vi "TSM SSC DAQmx Configure Sync Pulse Source PXI Trig.vi"(0 "DAQ TSM in":T1, 5 "source(PXI_Trig0)":string(combo)="PXI_Trig0", 11 "error in (no error)":errorcluster) -> (4 "DAQ TSM Out":T1, 15 "error out":errorcluster)   [LabVIEW 2020]
doc: "Specifies the terminal of the signal to use as the synchronization pulse. The synchronization pulse resets the clock dividers and the ADCs/DACs on the device."
uses:
  Pin Map/TSM DAQmx Multi-Task.ctl
  <vilib>/NI_TestStand_SemiconductorModule/NI_TestStand_Semiconductor_Module.lvlibp/PinMap/PinQueryContext/MultiplePinMultipleSessionQueryContext/MultiplePinMultipleSessionQueryContext.lvclass
  Pin Map/SSC DAQmx.ctl
  <resource>/objmgr/daqmx.rc
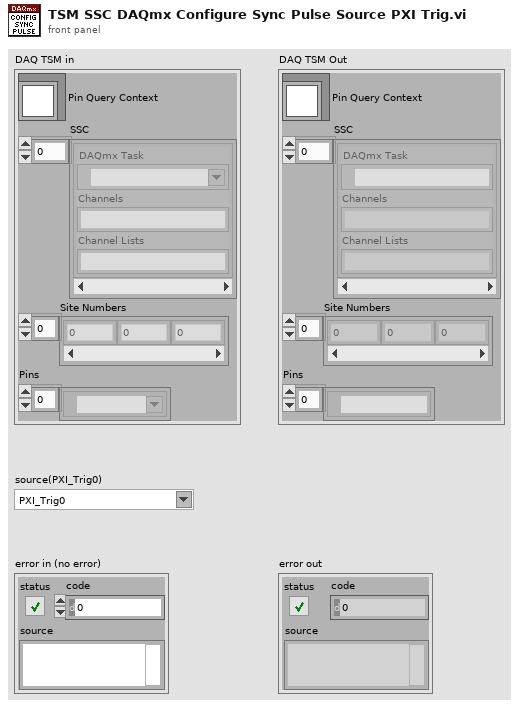
[diagram p1: front panel]
types:
  T1 = typedef "TSM DAQmx Multi-Task.ctl" = cluster{"Pin Query Context":refnum<class "MultiplePinMultipleSessionQueryContext.lvclass">, "SSC":T2[], "Site Numbers":i32[], "Pins":tag[]}
  T2 = typedef "SSC DAQmx.ctl" = cluster{"DAQmx Task ":refnum<k21>, "Channels":string, "Channel Lists":string}
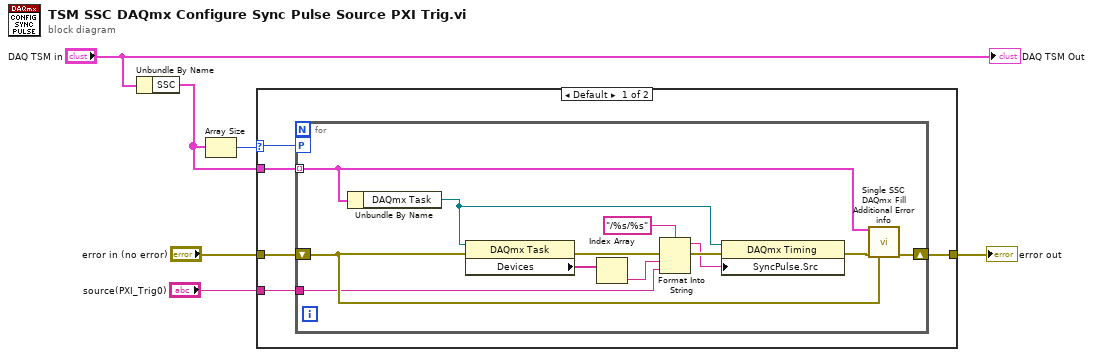
[diagram p0: block diagram]
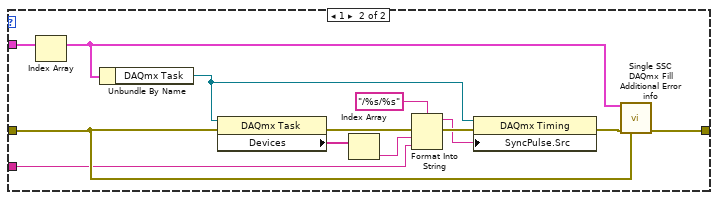
[diagram p2: hidden frame]
diagram:
  n1 = Unbundle By Name("DAQ TSM in") -> ("SSC"=w4:T2[])
  n2 = Array Size(array=w4) -> (size(s)=w5:i32)
  n3 = case shown="Default" w5 {
    selector: w5 -> [w9 _]
    tunnel: [w11 w36] -> w2
    tunnel: "error in (no error)" -> [w10 w35]
    tunnel: w4 -> [w8 w34]
    tunnel: "source(PXI_Trig0)" -> [w7 w33]
    frame Default {
      n4 = for {
        tunnel: w8 -> [w22] mode=indexing
        workers-P: w9 -> [_]
        shift-right: [w23] -> w11
        shift-left: w10 -> [w21]
        tunnel: w7 -> [w14]
        n5 = Unbundle By Name(w22) -> ("DAQmx Task"=w18:refnum<k21>)
        n6 = property class="DAQmx Task"(reference=w18, error in=w21) -> (error out=w19:errorcluster, "Devices"=w16:tag[])  [unwired: 1 out]
        n7 = Index Array(array=w16) -> (element=w15:tag)  [unwired: 1 in]
        n8 = Format Into String(format string="/%s/%s", error in=w19, w15, w14) -> (resulting string=w12:string, error out=w17:errorcluster)  [unwired: 1 in]
        n9 = property class="DAQmx Timing"(reference=w18, error in=w17, "SyncPulse.Src"=w12) -> (error out=w20:errorcluster)  [unwired: 1 out]
        n10 = call "Single SSC DAQmx Fill Additional Error info.vi"("DAQmx SSC in"=w22, "error in"=w20, "previous error in"=w21) -> ("error out"=w23:errorcluster)  [unwired: 12 in]
      }
    }
    frame 1 {
      n11 = Index Array(array=w34) -> (element=w24:T2)  [unwired: 1 in]
      n12 = Unbundle By Name(w24) -> ("DAQmx Task"=w30:refnum<k21>)
      n13 = property class="DAQmx Task"(reference=w30, error in=w35) -> (error out=w31:errorcluster, "Devices"=w28:tag[])  [unwired: 1 out]
      n14 = Index Array(array=w28) -> (element=w27:tag)  [unwired: 1 in]
      n15 = Format Into String(format string="/%s/%s", error in=w31, w27, w33) -> (resulting string=w25:string, error out=w29:errorcluster)  [unwired: 1 in]
      n16 = property class="DAQmx Timing"(reference=w30, error in=w29, "SyncPulse.Src"=w25) -> (error out=w32:errorcluster)  [unwired: 1 out]
      n17 = call "Single SSC DAQmx Fill Additional Error info.vi"("DAQmx SSC in"=w24, "error in"=w32, "previous error in"=w35) -> ("error out"=w36:errorcluster)  [unwired: 12 in]
    }
  }
  "error out" <- w2
  "DAQ TSM Out" <- "DAQ TSM in"
